vi "Day 5.1 - .vi"(11 "input":string[](array[string])) -> (3 "output":string)   [LabVIEW 2021]
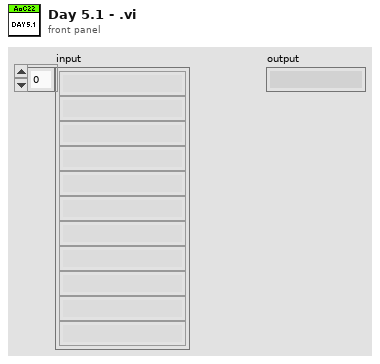
[diagram p1: front panel]
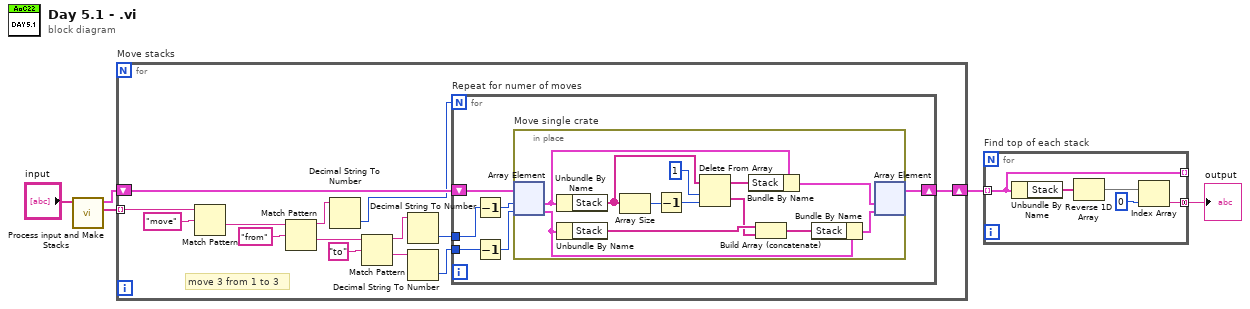
[diagram p0: block diagram]
diagram:
  n1 = call "Process input and Make Stacks.vi"("input"="input") -> ("Moves"=w3:string[], "Stacks"=w2:cluster{"Label":string, "Stack":string[]}[])  [unwired: 9 in]
  n2 = for "Move stacks" {
    tunnel: w3 -> [w19] mode=indexing
    shift-right: [w6] -> w1
    shift-left: w2 -> [w10]
    # "move 3 from 1 to 3"
    n3 = Match Pattern(string=w19, regular expression="move") -> (after substring=w17:string)  [unwired: 1 in, 3 out]
    n4 = Match Pattern(string=w17, regular expression="from") -> (before substring=w13:string, after substring=w15:string)  [unwired: 1 in, 2 out]
    n5 = Decimal String To Number(string=w13) -> (number=w9:i32)  [unwired: 2 in, 1 out]
    n6 = Match Pattern(string=w15, regular expression="to") -> (before substring=w12:string, after substring=w11:string)  [unwired: 1 in, 2 out]
    n7 = Decimal String To Number(string=w12) -> (number=w8:i32)  [unwired: 2 in, 1 out]
    n8 = Decimal String To Number(string=w11) -> (number=w7:i32)  [unwired: 2 in, 1 out]
    n9 = for "Repeat for numer of moves" {
      N: w9 -> [_]
      tunnel: w8 -> [w24]
      shift-right: [w22] -> w6
      shift-left: w10 -> [w25]
      tunnel: w7 -> [w23]
      n10 = Decrement(x=w24) -> (x-1=w21:i32)
      n11 = Decrement(x=w23) -> (x-1=w20:i32)
      n12 = in-place "Move single crate" {
        n13 = in-place-array #1(w25, w21, w20) -> (w36:cluster{"Label":string, "Stack":string[]}, w34:cluster{"Label":string, "Stack":string[]})
        n14 = Unbundle By Name(w36) -> ("Stack"=w33:string[])
        n15 = Unbundle By Name(w34) -> ("Stack"=w28:string[])
        n16 = Array Size(array=w33) -> (size(s)=w32:i32)
        n17 = Decrement(x=w32) -> (x-1=w30:i32)
        n18 = Delete From Array(array=w33, length=1, index=w30) -> (deleted portion=w27:string[], array with subset deleted=w29:string[])
        n19 = Bundle By Name(cluster=w36, "Stack"=w29) -> (w37:cluster{"Label":string, "Stack":string[]})
        n20 = Build Array (concatenate)(w28, w27) -> (w26:string[])
        n21 = Bundle By Name(cluster=w34, "Stack"=w26) -> (w35:cluster{"Label":string, "Stack":string[]})
        n22 = in-place-array #1(w37, w35) -> (w22:cluster{"Label":string, "Stack":string[]}[])  [unwired: 2 out]
      }
    }
  }
  n23 = for "Find top of each stack" {
    tunnel: [w38] -> _ mode=indexing
    tunnel: [w39] -> w4 mode=concatenating
    tunnel: w1 -> [w38] mode=indexing
    n24 = Unbundle By Name(w38) -> ("Stack"=w42:string[])
    n25 = Reverse 1D Array(array=w42) -> (reversed array=w41:string[])
    n26 = Index Array(array=w41, index=0) -> (element=w39:string)
  }
  "output" <- w4
